vi "Laser Controller.vi"(8 "error in (no error)":errorcluster, 10 "Notifiers":T1, 11 "All Message Queue Cluster":T2) -> (0 "error out":errorcluster)   [LabVIEW 2017]
uses:
  Lib QMH/AllMessageQueue Cluster.ctl
  Lib QMH/Message Cluster.ctl
  Lib Notifier/Notifier.ctl
  Lib QMH/MessageQueues.lvlib
  Lib Log/Logging.lvlib
  Lib Notifier/Notifier.lvlib
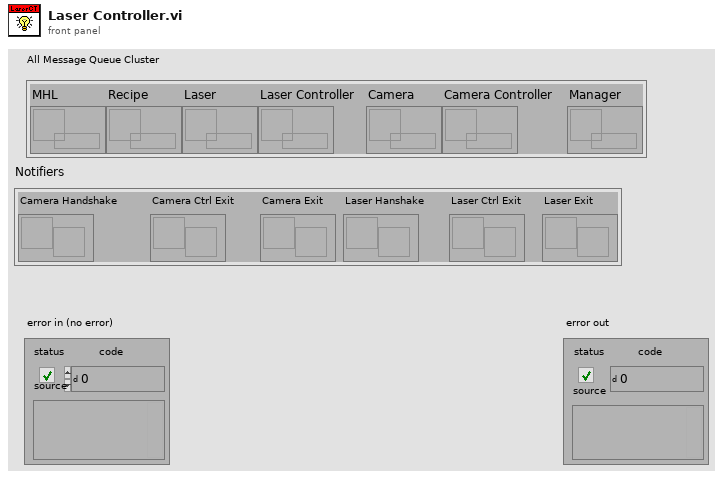
[diagram p1: front panel]
types:
  T1 = typedef "Notifier.lvlib/Notifier.ctl" = cluster{"Camera Handshake":refnum<notifier>, "Camera Ctrl Exit":refnum<notifier>, "Camera Exit":refnum<notifier>, "Laser Hanshake":refnum<notifier>, "Laser Ctrl Exit":refnum<notifier>, "Laser Exit":refnum<notifier>}
  T2 = typedef "MessageQueues.lvlib/AllMessageQueue Cluster.ctl" = cluster{"MHL":refnum<queue>, "Recipe":refnum<queue>, "Laser":refnum<queue>, "Laser Controller":refnum<queue>, "Camera":refnum<queue>, "Camera Controller":refnum<queue>, "Manager":refnum<queue>}
  T3 = enum16{"open", "replace", "create", "open or create", "replace or create", "replace or create with confirmation"}
  T4 = cluster{"état":bool, "code":i32, "source":string}
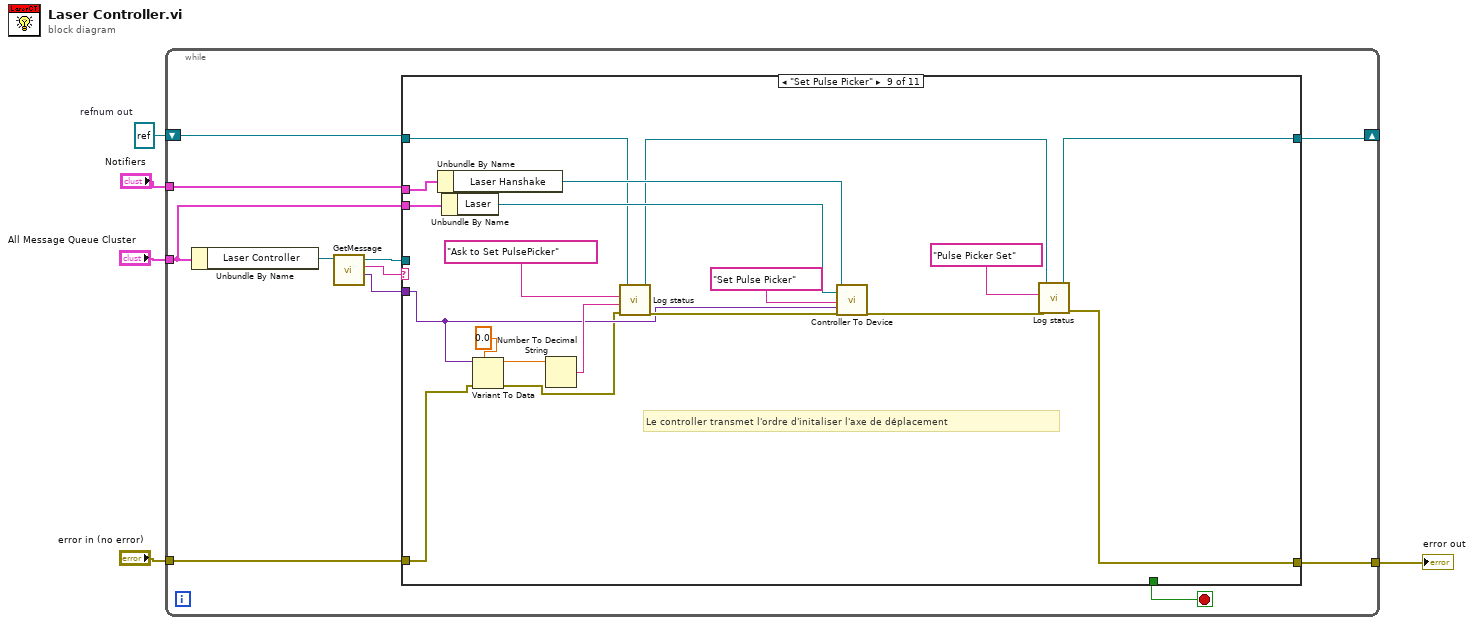
[diagram p0: block diagram]
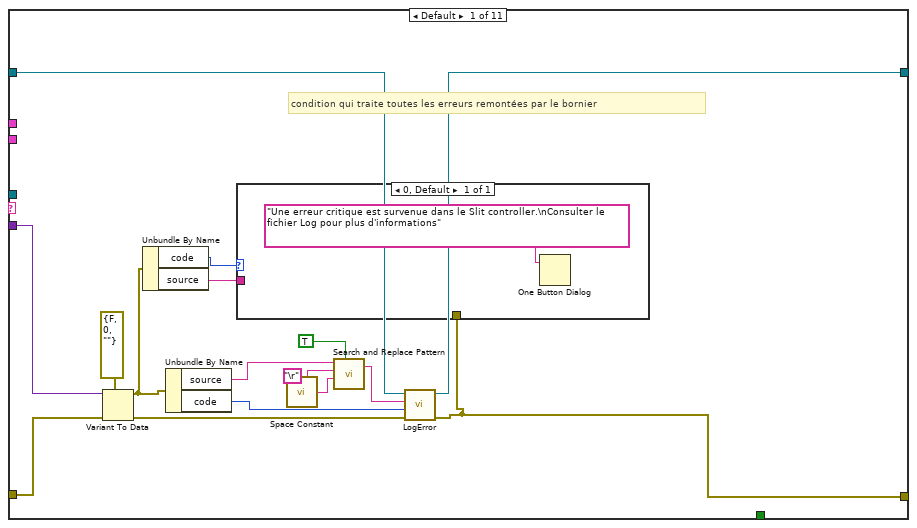
[diagram p2: hidden frame]
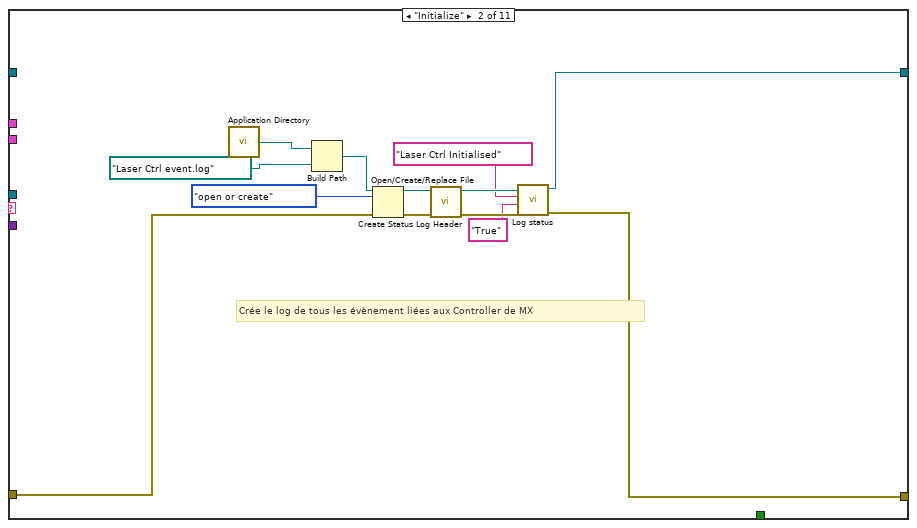
[diagram p3: hidden frame]
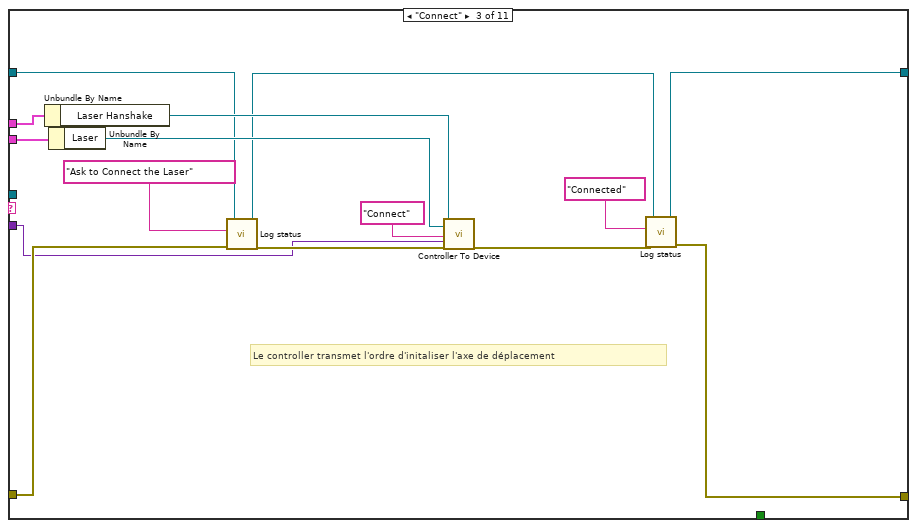
[diagram p4: hidden frame]
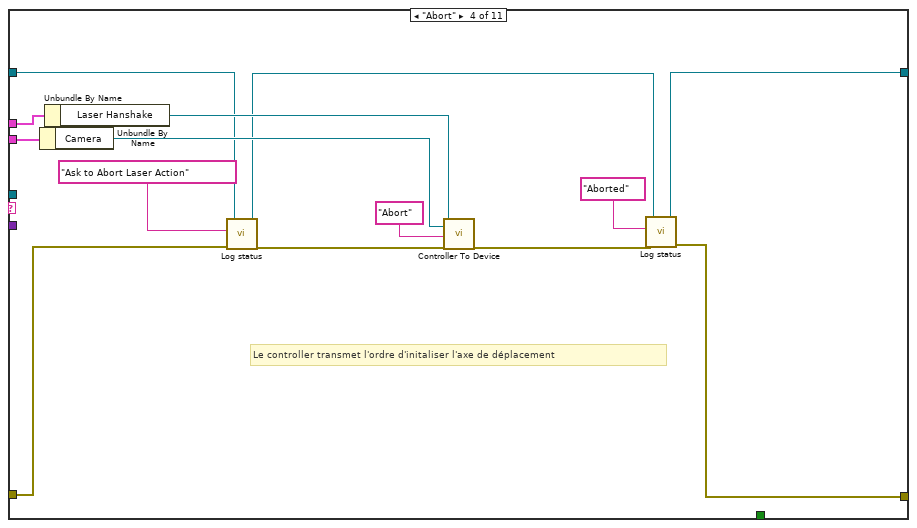
[diagram p5: hidden frame]
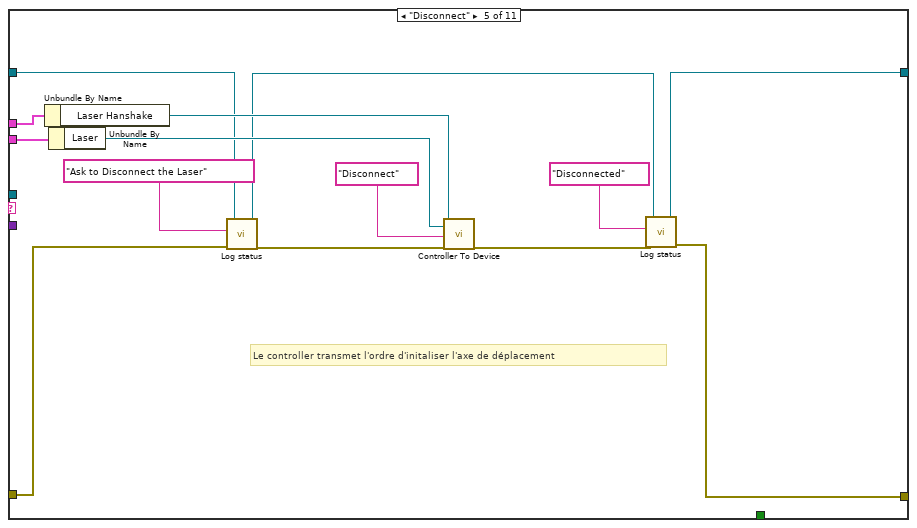
[diagram p6: hidden frame]
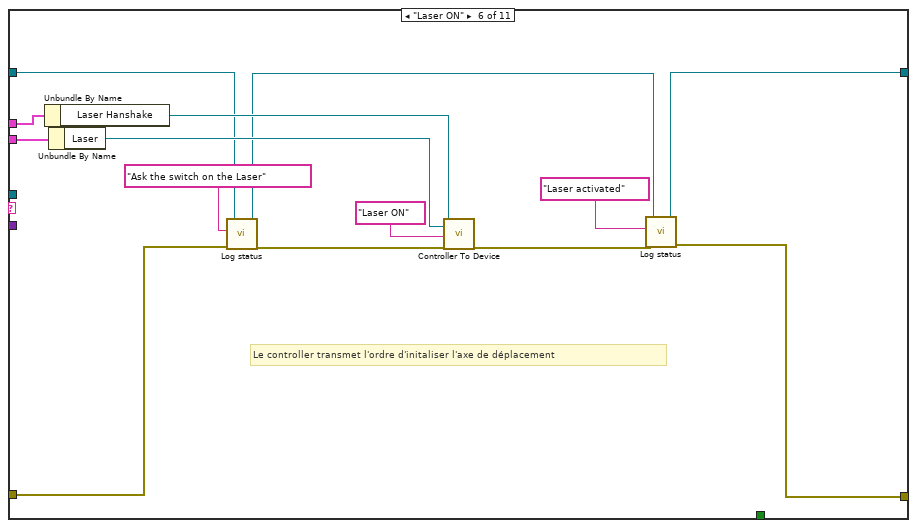
[diagram p7: hidden frame]
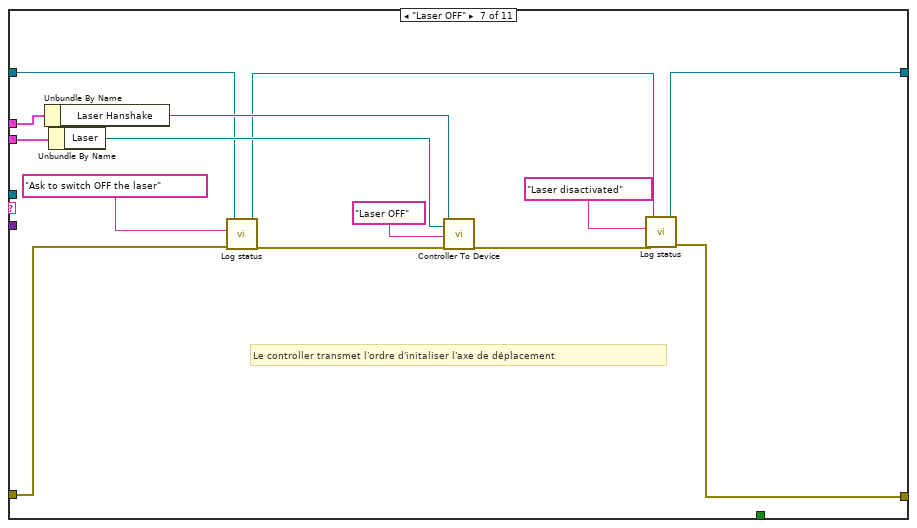
[diagram p8: hidden frame]
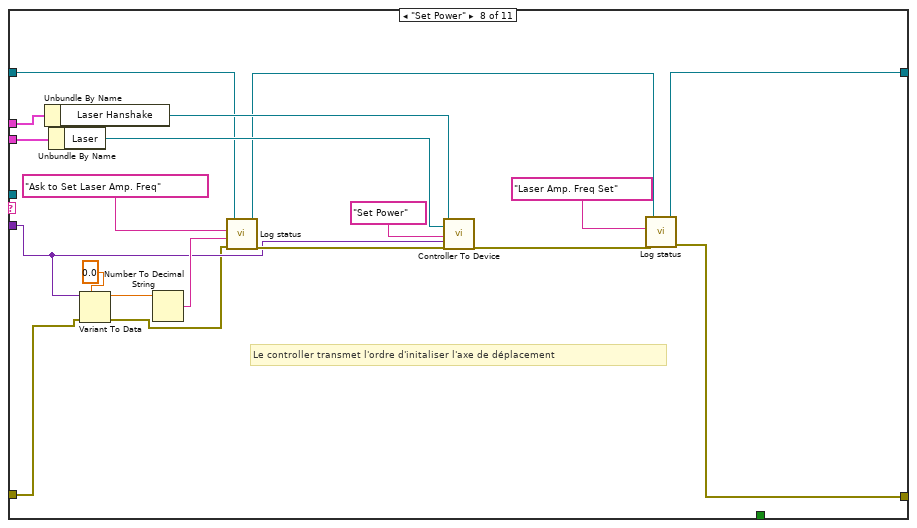
[diagram p9: hidden frame]
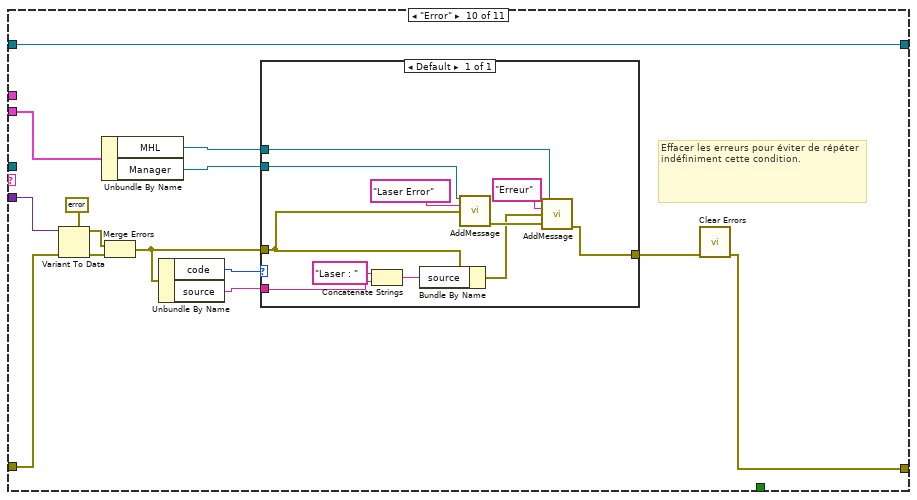
[diagram p10: hidden frame]
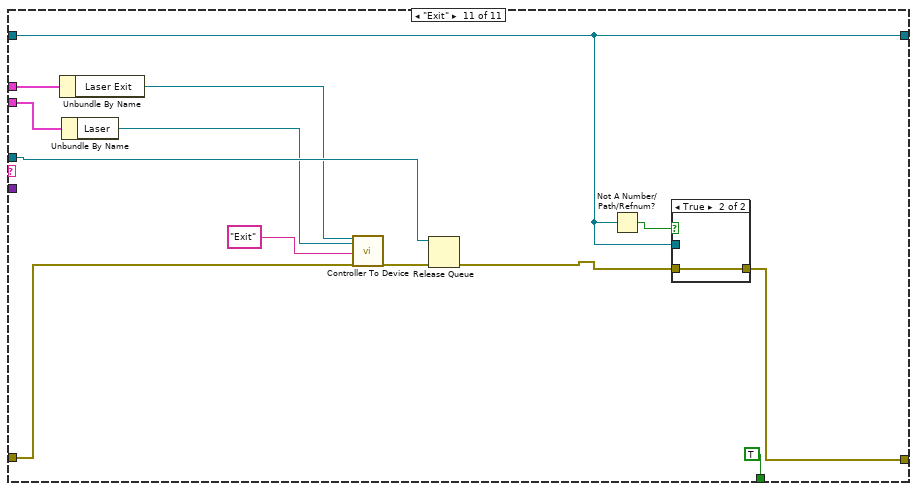
[diagram p11: hidden frame]
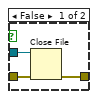
[diagram p12: hidden frame]
diagram:
  w2 = refnum<file> refnum  # refnum out
  n1 = while {
    tunnel: "All Message Queue Cluster" -> [w10]
    tunnel: "Notifiers" -> [w9]
    tunnel: "error in (no error)" -> [w8]
    tunnel: [w15] -> w1
    shift-right: [w12] -> _
    shift-left: w2 -> [w13]
    stop <- w14 stop-if-true
    n2 = Unbundle By Name(w10) -> ("Laser Controller"=w16:refnum<queue>)
    n3 = call "GetMessage.vi"("Message queue"=w16) -> ("Data"=w7:variant, "Message"=w6:string, "Dup Message Queue"=w11:refnum<queue>)  [unwired: 7 in, 1 out]
    n4 = case shown="\"Set Pulse Picker\"" w6 {
      tunnel: w9 -> [_ _ w61 w75 w89 w103 w117 w136 w155 _ w190]
      tunnel: w10 -> [_ _ w60 w74 w88 w102 w116 w135 w154 w158 w189]
      tunnel: w8 -> [w21 w36 w49 w63 w77 w91 w105 w119 w138 w160 w185]
      tunnel: [_ _ _ _ _ _ _ _ _ _ TRUE] -> w14
      tunnel: w11 -> [_ _ _ _ _ _ _ _ _ _ w191]
      tunnel: w7 -> [w19 _ w47 _ _ _ _ w120 w139 w161 _]
      tunnel: [w17 w34 w52 w66 w80 w94 w108 w127 w146 w169 w187] -> w12
      tunnel: w13 -> [w18 _ w56 w70 w84 w98 w112 w131 w150 w169 w187]
      tunnel: [w20 w35 w54 w68 w82 w96 w110 w129 w148 w159 w188] -> w15
      frame Default {
        # "condition qui traite toutes les erreurs remontées par le bornier"
        n5 = Variant To Data(error in=w21, type=errorcluster {"status"=FALSE, "code"=0, "source"=""} ("error in (no error)"), Variant=w19) -> (data=w32:errorcluster, error out=w23:errorcluster)
        n6 = Unbundle By Name(w32) -> ("code"=w30:i32, "source"=w31:string)
        n7 = Unbundle By Name(w32) -> ("source"=w25:string, "code"=w24:i32)
        n8 = call <vilib>:"Space Constant.vi"() -> ("String"=w27:string)
        n9 = call <vilib>:"Search and Replace Pattern.vi"("string"=w25, "regular expression (\"\")"="\r", "replace string (\"\")"=w27, "replace all? (F)"=TRUE) -> ("result string"=w28:string)  [unwired: 1 in, 1 out]
        n10 = call "LogError.vi"("entrée d'erreur"=w23, "Code"=w24, "Source"=w28, "Error log refnum In"=w18) -> ("error out"=w20:errorcluster, "Error log refnum out"=w17:refnum<file>)  [unwired: 6 in]
        n11 = case shown="0, Default" w30 {
          tunnel: w31 -> [_]
          tunnel: w20 -> [_]
          frame 0, Default {
            n12 = One Button Dialog(message="Une erreur critique est survenue dans le Slit controller.\nConsulter le fichier Log pour plus d'informations" ("chaîne de format")) -> ()  [unwired: 1 in, 1 out]
          }
        }
      }
      frame "Initialize" {
        # "Crée le log de tous les évènement liées aux Controller de MX"
        n13 = call <vilib>:"Application Directory.vi"() -> ("Application Directory"=w43:path)
        n14 = Build Path(base path=w43, name or relative path=path "Laser Ctrl event.log") -> (appended path=w45:path)
        n15 = Open/Create/Replace File(file path (use dialog)=w45, error in=w36, operation (0:open)=T3."open or create" ("opération (0 : open)")) -> (refnum out=w41:refnum<file>, error out=w42:errorcluster)  [unwired: 3 in, 1 out]
        n16 = call "Create Status Log Header.vi"("entrée d'erreur"=w42, "Log File Refnum In"=w41) -> ("sortie d'erreur"=w40:errorcluster, "Log File Refnum out"=w39:refnum<file>)  [unwired: 8 in]
        n17 = call "Log status.vi"("entrée d'erreur"=w40, "Event Data String (-)"="True", "Event string"="Laser Ctrl Initialised", "Log File Refnum In"=w39) -> ("error out"=w35:errorcluster, "Log File Refnum out"=w34:refnum<file>)  [unwired: 6 in]
      }
      frame "Connect" {
        # "Le controller transmet l'ordre d'initaliser l'axe de déplacement"
        n18 = Unbundle By Name(w61) -> ("Laser Hanshake"=w59:refnum<notifier>)
        n19 = Unbundle By Name(w60) -> ("Laser"=w58:refnum<queue>)
        n20 = call "Log status.vi"("entrée d'erreur"=w49, "Event string"="Ask to Connect the Laser", "Log File Refnum In"=w56) -> ("error out"=w57:errorcluster, "Log File Refnum out"=w53:refnum<file>)  [unwired: 7 in]
        n21 = call "Controller To Device.vi"("Notifier"=w59, "Message queue"=w58, "Message"="Connect", "Data"=w47, "entrée d'erreur"=w57) -> ("sortie d'erreur"=w55:errorcluster)  [unwired: 12 in, 2 out]
        n22 = call "Log status.vi"("entrée d'erreur"=w55, "Event string"="Connected", "Log File Refnum In"=w53) -> ("error out"=w54:errorcluster, "Log File Refnum out"=w52:refnum<file>)  [unwired: 7 in]
      }
      frame "Abort" {
        # "Le controller transmet l'ordre d'initaliser l'axe de déplacement"
        n23 = Unbundle By Name(w74) -> ("Camera"=w72:refnum<queue>)
        n24 = Unbundle By Name(w75) -> ("Laser Hanshake"=w73:refnum<notifier>)
        n25 = call "Log status.vi"("entrée d'erreur"=w63, "Event string"="Ask to Abort Laser Action", "Log File Refnum In"=w70) -> ("error out"=w71:errorcluster, "Log File Refnum out"=w67:refnum<file>)  [unwired: 7 in]
        n26 = call "Controller To Device.vi"("Notifier"=w73, "Message queue"=w72, "Message"="Abort", "entrée d'erreur"=w71) -> ("sortie d'erreur"=w69:errorcluster)  [unwired: 13 in, 2 out]
        n27 = call "Log status.vi"("entrée d'erreur"=w69, "Event string"="Aborted", "Log File Refnum In"=w67) -> ("error out"=w68:errorcluster, "Log File Refnum out"=w66:refnum<file>)  [unwired: 7 in]
      }
      frame "Disconnect" {
        # "Le controller transmet l'ordre d'initaliser l'axe de déplacement"
        n28 = Unbundle By Name(w89) -> ("Laser Hanshake"=w87:refnum<notifier>)
        n29 = Unbundle By Name(w88) -> ("Laser"=w86:refnum<queue>)
        n30 = call "Log status.vi"("entrée d'erreur"=w77, "Event string"="Ask to Disconnect the Laser", "Log File Refnum In"=w84) -> ("error out"=w85:errorcluster, "Log File Refnum out"=w81:refnum<file>)  [unwired: 7 in]
        n31 = call "Controller To Device.vi"("Notifier"=w87, "Message queue"=w86, "Message"="Disconnect", "entrée d'erreur"=w85) -> ("sortie d'erreur"=w83:errorcluster)  [unwired: 13 in, 2 out]
        n32 = call "Log status.vi"("entrée d'erreur"=w83, "Event string"="Disconnected", "Log File Refnum In"=w81) -> ("error out"=w82:errorcluster, "Log File Refnum out"=w80:refnum<file>)  [unwired: 7 in]
      }
      frame "Laser ON" {
        # "Le controller transmet l'ordre d'initaliser l'axe de déplacement"
        n33 = Unbundle By Name(w103) -> ("Laser Hanshake"=w101:refnum<notifier>)
        n34 = Unbundle By Name(w102) -> ("Laser"=w100:refnum<queue>)
        n35 = call "Log status.vi"("entrée d'erreur"=w91, "Event string"="Ask the switch on the Laser", "Log File Refnum In"=w98) -> ("error out"=w99:errorcluster, "Log File Refnum out"=w95:refnum<file>)  [unwired: 7 in]
        n36 = call "Controller To Device.vi"("Notifier"=w101, "Message queue"=w100, "Message"="Laser ON", "entrée d'erreur"=w99) -> ("sortie d'erreur"=w97:errorcluster)  [unwired: 13 in, 2 out]
        n37 = call "Log status.vi"("entrée d'erreur"=w97, "Event string"="Laser activated", "Log File Refnum In"=w95) -> ("error out"=w96:errorcluster, "Log File Refnum out"=w94:refnum<file>)  [unwired: 7 in]
      }
      frame "Laser OFF" {
        # "Le controller transmet l'ordre d'initaliser l'axe de déplacement"
        n38 = Unbundle By Name(w117) -> ("Laser Hanshake"=w115:refnum<notifier>)
        n39 = Unbundle By Name(w116) -> ("Laser"=w114:refnum<queue>)
        n40 = call "Log status.vi"("entrée d'erreur"=w105, "Event string"="Ask to switch OFF the laser", "Log File Refnum In"=w112) -> ("error out"=w113:errorcluster, "Log File Refnum out"=w109:refnum<file>)  [unwired: 7 in]
        n41 = call "Controller To Device.vi"("Notifier"=w115, "Message queue"=w114, "Message"="Laser OFF", "entrée d'erreur"=w113) -> ("sortie d'erreur"=w111:errorcluster)  [unwired: 13 in, 2 out]
        n42 = call "Log status.vi"("entrée d'erreur"=w111, "Event string"="Laser disactivated", "Log File Refnum In"=w109) -> ("error out"=w110:errorcluster, "Log File Refnum out"=w108:refnum<file>)  [unwired: 7 in]
      }
      frame "Set Power" {
        # "Le controller transmet l'ordre d'initaliser l'axe de déplacement"
        n43 = Unbundle By Name(w136) -> ("Laser Hanshake"=w134:refnum<notifier>)
        n44 = Unbundle By Name(w135) -> ("Laser"=w133:refnum<queue>)
        n45 = Variant To Data(error in=w119, type=0.0, Variant=w120) -> (data=w122:dbl, error out=w118:errorcluster)
        n46 = Number To Decimal String(number=w122) -> (decimal integer string=w121:string)  [unwired: 1 in]
        n47 = call "Log status.vi"("entrée d'erreur"=w118, "Event Data String (-)"=w121, "Event string"="Ask to Set Laser Amp. Freq", "Log File Refnum In"=w131) -> ("error out"=w132:errorcluster, "Log File Refnum out"=w128:refnum<file>)  [unwired: 6 in]
        n48 = call "Controller To Device.vi"("Notifier"=w134, "Message queue"=w133, "Message"="Set Power", "Data"=w120, "entrée d'erreur"=w132) -> ("sortie d'erreur"=w130:errorcluster)  [unwired: 12 in, 2 out]
        n49 = call "Log status.vi"("entrée d'erreur"=w130, "Event string"="Laser Amp. Freq Set", "Log File Refnum In"=w128) -> ("error out"=w129:errorcluster, "Log File Refnum out"=w127:refnum<file>)  [unwired: 7 in]
      }
      frame "Set Pulse Picker" {
        # "Le controller transmet l'ordre d'initaliser l'axe de déplacement"
        n50 = Unbundle By Name(w155) -> ("Laser Hanshake"=w153:refnum<notifier>)
        n51 = Unbundle By Name(w154) -> ("Laser"=w152:refnum<queue>)
        n52 = Variant To Data(error in=w138, type=0.0, Variant=w139) -> (data=w141:dbl, error out=w137:errorcluster)
        n53 = Number To Decimal String(number=w141) -> (decimal integer string=w140:string)  [unwired: 1 in]
        n54 = call "Log status.vi"("entrée d'erreur"=w137, "Event Data String (-)"=w140, "Event string"="Ask to Set PulsePicker", "Log File Refnum In"=w150) -> ("error out"=w151:errorcluster, "Log File Refnum out"=w147:refnum<file>)  [unwired: 6 in]
        n55 = call "Controller To Device.vi"("Notifier"=w153, "Message queue"=w152, "Message"="Set Pulse Picker", "Data"=w139, "entrée d'erreur"=w151) -> ("sortie d'erreur"=w149:errorcluster)  [unwired: 12 in, 2 out]
        n56 = call "Log status.vi"("entrée d'erreur"=w149, "Event string"="Pulse Picker Set", "Log File Refnum In"=w147) -> ("error out"=w148:errorcluster, "Log File Refnum out"=w146:refnum<file>)  [unwired: 7 in]
      }
      frame "Error" {
        # "Effacer les erreurs pour éviter de répéter indéfiniment cette condition."
        n57 = Variant To Data(error in=w160, type=T4 {"état"=FALSE, "code"=0, "source"=""} ("sortie d'erreur"), Variant=w161) -> (data=w166:T4, error out=w167:errorcluster)
        n58 = Unbundle By Name(w158) -> ("MHL"=w157:refnum<queue>, "Manager"=w162:refnum<queue>)
        n59 = Merge Errors(w166, w167) -> (w163:errorcluster)
        n60 = Unbundle By Name(w163) -> ("code"=w164:i32, "source"=w156:string)
        n61 = case shown="Default" w164 {
          tunnel: [w178] -> w165
          tunnel: w163 -> [w171]
          tunnel: w162 -> [w175]
          tunnel: w157 -> [w176]
          tunnel: w156 -> [w172]
          frame Default {
            n62 = Concatenate Strings("Laser : " ("string"), w172) -> (w173:string)
            n63 = Bundle By Name(cluster=w171, "source"=w173) -> (w170:errorcluster)
            n64 = call "AddMessage.vi"("Message queue"=w175, "Message"="Laser Error", "Data"=w171) -> ("error out"=w177:errorcluster)  [unwired: 11 in, 1 out]
            n65 = call "AddMessage.vi"("Message queue"=w176, "Message"="Erreur", "Data"=w170, "entrée d'erreur (pas d'erreur)"=w177) -> ("error out"=w178:errorcluster)  [unwired: 10 in, 1 out]
          }
        }
        n66 = call <vilib>:"Clear Errors.vi"("error in (no error)"=w165) -> ("error out"=w159:errorcluster)  [unwired: 5 in, 1 out]
      }
      frame "Exit" {
        n67 = Unbundle By Name(w190) -> ("Laser Exit"=w183:refnum<notifier>)
        n68 = Unbundle By Name(w189) -> ("Laser"=w182:refnum<queue>)
        n69 = call "Controller To Device.vi"("Notifier"=w183, "Message queue"=w182, "Message"="Exit", "entrée d'erreur"=w185) -> ("sortie d'erreur"=w186:errorcluster)  [unwired: 13 in, 2 out]
        n70 = Release Queue(queue=w191, error in (no error)=w186) -> (error out=w181:errorcluster)  [unwired: 1 in, 2 out]
        n71 = Not A Number/Path/Refnum?(number/path/refnum=w187) -> (NaN/Path/Refnum?=w192:bool)
        n72 = case shown="True" w192 {
          tunnel: [w196 w197] -> w188
          tunnel: w181 -> [w195 w197]
          tunnel: w187 -> [w194 _]
          frame False {
            n73 = Close File(refnum=w194, error in=w195) -> (error out=w196:errorcluster)  [unwired: 1 out]
          }
          frame True {
          }
        }
      }
    }
  }
  "error out" <- w1
